vi "Depth Frame Read.vi"(8 "error in (no error)":errorcluster, 11 "Video Frame in":refnum<class "Video Frame.lvclass">) -> (0 "error out":errorcluster, 2 "Depth Values":dbl[](array[numeric]), 3 "Video Frame out":refnum<class "Video Frame.lvclass">, 4 "Average Depth":dbl, 6 "Standard Deviation":dbl)   [LabVIEW 2018, in "Video Frame.lvclass"]
uses:
  Video Frame.lvclass
  Video Frame.lvclass/Video Frame.ctl
  52481fbb-3c2e-4496-a16e-d7e242c0092f.vi
  3d6fd04e-ddc9-4726-8c48-280292d52a2f.vi
  3bcc8776-fff3-4aac-9a6b-1c6d02c9ff80.vi
  3bcc8776-fff3-4aac-9a6b-1c6d02c9ff80.vi/82d6821c-224f-4e7a-bda4-0c0196720146.vi
  <vilib>/vision/NI_Vision_Development_Module.lvlib
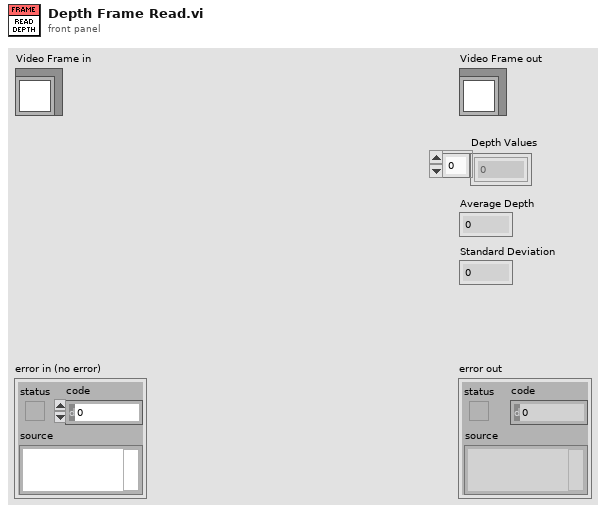
[diagram p1: front panel]
types:
  T1 = typedef "IMAQ Image.ctl" = refnum<image>
  T2 = typedef "Image Type" = u32
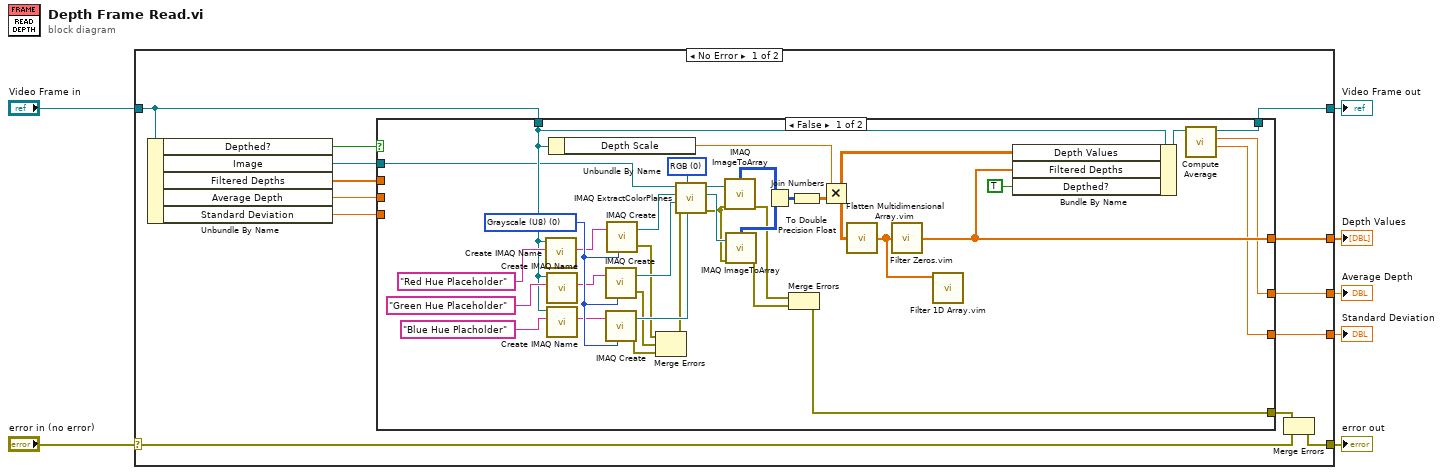
[diagram p0: block diagram]
diagram:
  n1 = case shown="No Error" "error in (no error)" {
    selector: "error in (no error)" -> [w9 w62]
    tunnel: [w8 w62] -> w6
    tunnel: [w17 w61] -> w4
    tunnel: "Video Frame in" -> [w16 w61]
    tunnel: [w15 _] -> w3
    tunnel: [w14 _] -> w2
    tunnel: [w13 _] -> w1
    frame No Error {
      n2 = Unbundle By Name(w16) -> ("Depthed?"=w12:bool, "Image"=w11:T1, "Filtered Depths"=w20:dbl[], "Average Depth"=w19:dbl, "Standard Deviation"=w18:dbl)
      n3 = case shown="False" w12 {
        tunnel: w16 -> [w38 w60]
        tunnel: w20 -> [_ w59]
        tunnel: w19 -> [_ w58]
        tunnel: w18 -> [_ w57]
        tunnel: [w32 w60] -> w17
        tunnel: [w36 w59] -> w15
        tunnel: [w31 w58] -> w14
        tunnel: [w30 w57] -> w13
        tunnel: w11 -> [w37 _]
        tunnel: [w21 _] -> w10
        frame False {
          w46 = u16 0 items=["RGB", "HSL", "HSV", "HSI"] ("Color Mode")
          w53 = T2 0 items=["Grayscale (U8)", "Grayscale (I16)", "Grayscale (SGL)", "Complex (CSG)", "RGB (U32)", "HSL (U32)", "RGB (U64)", "Grayscale (U16)"] ("Image Type")
          n4 = call-dynamic "Create IMAQ Name.vi"("Name (\"\")"="Red Hue Placeholder" ("Image Name"), "Video Frame in"=w38) -> ("Name Out"=w52:string)  [unwired: 7 in, 2 out]
          n5 = call-dynamic "Create IMAQ Name.vi"("Name (\"\")"="Green Hue Placeholder" ("Image Name"), "Video Frame in"=w38) -> ("Name Out"=w51:string)  [unwired: 7 in, 2 out]
          n6 = call-dynamic "Create IMAQ Name.vi"("Name (\"\")"="Blue Hue Placholder" ("Image Name"), "Video Frame in"=w38) -> ("Name Out"=w50:string)  [unwired: 7 in, 2 out]
          n7 = Unbundle By Name(w38) -> ("Depth Scale"=w39:dbl)
          n8 = call "IMAQ Create"("Image Name"=w51, "Image Type"=w53) -> ("New Image"=w48:T1, "error out"=w26:errorcluster)  [unwired: 3 in]
          n9 = call "IMAQ Create"("Image Name"=w50, "Image Type"=w53) -> ("New Image"=w47:T1, "error out"=w27:errorcluster)  [unwired: 3 in]
          n10 = call "IMAQ Create"("Image Name"=w52, "Image Type"=w53) -> ("New Image"=w49:T1, "error out"=w25:errorcluster)  [unwired: 3 in]
          n11 = Merge Errors(w25, w26, w27) -> (w24:errorcluster)
          n12 = call "IMAQ ExtractColorPlanes"("Blue or Luma or Val or Inten Plane"=w47, "Color Mode"=w46, "error in (no error)"=w24, "Green or Sat Plane"=w48, "Red or Hue Plane"=w49, "Image Src"=w37) -> ("error out"=w28:errorcluster, "Green or Sat Plane out"=w44:T1, "Red or Hue Plane out"=w45:T1)  [unwired: 2 in, 1 out]
          n13 = call "IMAQ ImageToArray"("error in (no error)"=w28, "Image"=w45) -> ("error out"=w23:errorcluster, "Image Pixels (U8)"=w43:u8[][])  [unwired: 2 in, 3 out]
          n14 = call "IMAQ ImageToArray"("error in (no error)"=w28, "Image"=w44) -> ("error out"=w22:errorcluster, "Image Pixels (U8)"=w42:u8[][])  [unwired: 2 in, 3 out]
          n15 = Join Numbers(hi=w43, lo=w42) -> ((hi.lo)=w41:u16[][])
          n16 = Merge Errors(w23, w22) -> (w21:errorcluster)
          n17 = To Double Precision Float(number=w41) -> (double precision float=w40:dbl[][])
          n18 = Multiply(x=w39, y=w40) -> (x*y=w35:dbl[][])
          n19 = call "Flatten Multidimensional Array.vim"("Array"=w35) -> ("output array"=w29:dbl[])  [unwired: 14 in]
          n20 = call "Filter Zeros.vim"("Array"=w29) -> ("Array Out"=w36:dbl[])  [unwired: 14 in]
          n21 = call "Filter 1D Array.vim"("Array"=w29) -> ()  [unwired: 10 in, 1 out]
          n22 = Bundle By Name(cluster=w38, "Depth Values"=w35, "Filtered Depths"=w36, "Depthed?"=TRUE) -> (w33:refnum<class "Video Frame.lvclass">)
          n23 = call-dynamic "Compute Average.vi"("Video Frame in"=w33) -> ("Standard Deviation"=w30:dbl, "Average"=w31:dbl, "Video Frame out"=w32:refnum<class "Video Frame.lvclass">)  [unwired: 7 in, 1 out]
        }
        frame True {
        }
      }
      n24 = Merge Errors(w10, w9) -> (w8:errorcluster)
    }
    frame Error {
    }
  }
  "error out" <- w6
  "Video Frame out" <- w4
  "Depth Values" <- w3
  "Average Depth" <- w2
  "Standard Deviation" <- w1
